vi "SplitURLu-p.vi"(10 "url|u:p":string) -> (1 "URL":string, 2 "pasword":string, 3 "username":string)   [LabVIEW 2021]
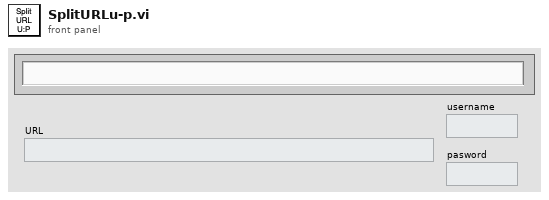
[diagram p1: front panel]
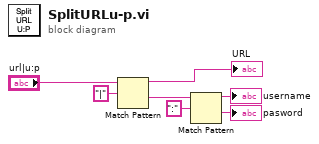
[diagram p0: block diagram]
diagram:
  n1 = Match Pattern(string="url|u:p", regular expression="|") -> (before substring=→"URL":string, after substring=w4:string)  [unwired: 1 in, 2 out]
  n2 = Match Pattern(string=w4, regular expression=":") -> (before substring=→"username":string, after substring=→"pasword":string)  [unwired: 1 in, 2 out]
